vi "Process_calibration_test.vi"() -> ()   [LabVIEW 2015]
uses:
  <vilib>/Analysis/5stat.llb/RMS (DBL).vi
  <vilib>/measure/madcrms.llb/Basic Averaged DC-RMS for 1 Chan.vi
  <vilib>/measure/maspectr.llb/FFT Spectrum (Mag-Phase) for 1 Chan.vi
  <vilib>/measure/NI_MAPro.lvlib
  <vilib>/Analysis/NI_AALPro.lvlib
  <vilib>/Analysis/NI_AALBase.lvlib
  <vilib>/Analysis/3filter.llb/Butterworth Filter (DBL).vi
  <vilib>/Analysis/3filter.llb/Filter Passband Type.ctl
panel:
  out "Waveform Graph 4":waveform(dbl)[](graph)
  out "Calibration\nparameter":dbl
  out "Sensivity\ncalibrated\nmV/g":dbl
  in  "Pattern\namplitude":dbl=1.02
  out "Array 8":bool[](array[boolean])
  out "Mean\nfrequency":dbl format="%0.2f"
  out "Main\nFrequency":dbl[](array[numeric])
  out "Valid\nmeasur\nfrequency":bool[](array[boolean])
  out "max value 3":dbl
  out "max value 2":dbl
  out "x/y 2":dbl
  out "x/y":dbl
  out "max value":dbl
  out "max index(es)":i32
  out "df":dbl
  out "magnitude":dbl[](array[numeric])
  out "Waveform Graph 3":T1(graph)
  out "Array 7":dbl[](array[numeric])
  out "Array 6":bool[][](array[boolean])
  out "mV":dbl[][](array[numeric])
  out "Valid \nmeasurements":sgl[][](array[numeric])
  out "Valid index":dbl format="%0.2f"
  out "Array 5":bool[](array[boolean])
  out "x > y?":bool
  out "concatenated string":string
  out "Index\ninvalid":i32[](array[numeric])
  out "Valid\nindex 2":i32[](array[numeric])
  out "Nº meas.":i32
  out "Valid\nindex":i32[](array[numeric])
  out "Array 4":bool[](array[boolean])
  out "Array 2":i32[][](array[numeric])
  out "Array 3":i32[](array[numeric])
  out "All Files in Dir":path[](array[path])
  out "Array":bool[][](array[boolean])
  in  "Frecuencia\nmuestreo":dbl=25600.0
  in  "Pattern frequency (Hz)":dbl=159.2
  in  "Nº canales":i32=10
  out "Waveform Graph":waveform(dbl)[](graph)
  in  "Folder Path":path
  out "error out":errorcluster
  # "Min"
  # "Median"
  # "Mean"
  # "Variance"
  # "Max"
  # "G:\\Mi unidad\\WRD\\SERVICIOS_Disco_duro\\Euskotren\\Lugaritz\\2016-05\\Calibracion\\4D\\verde"
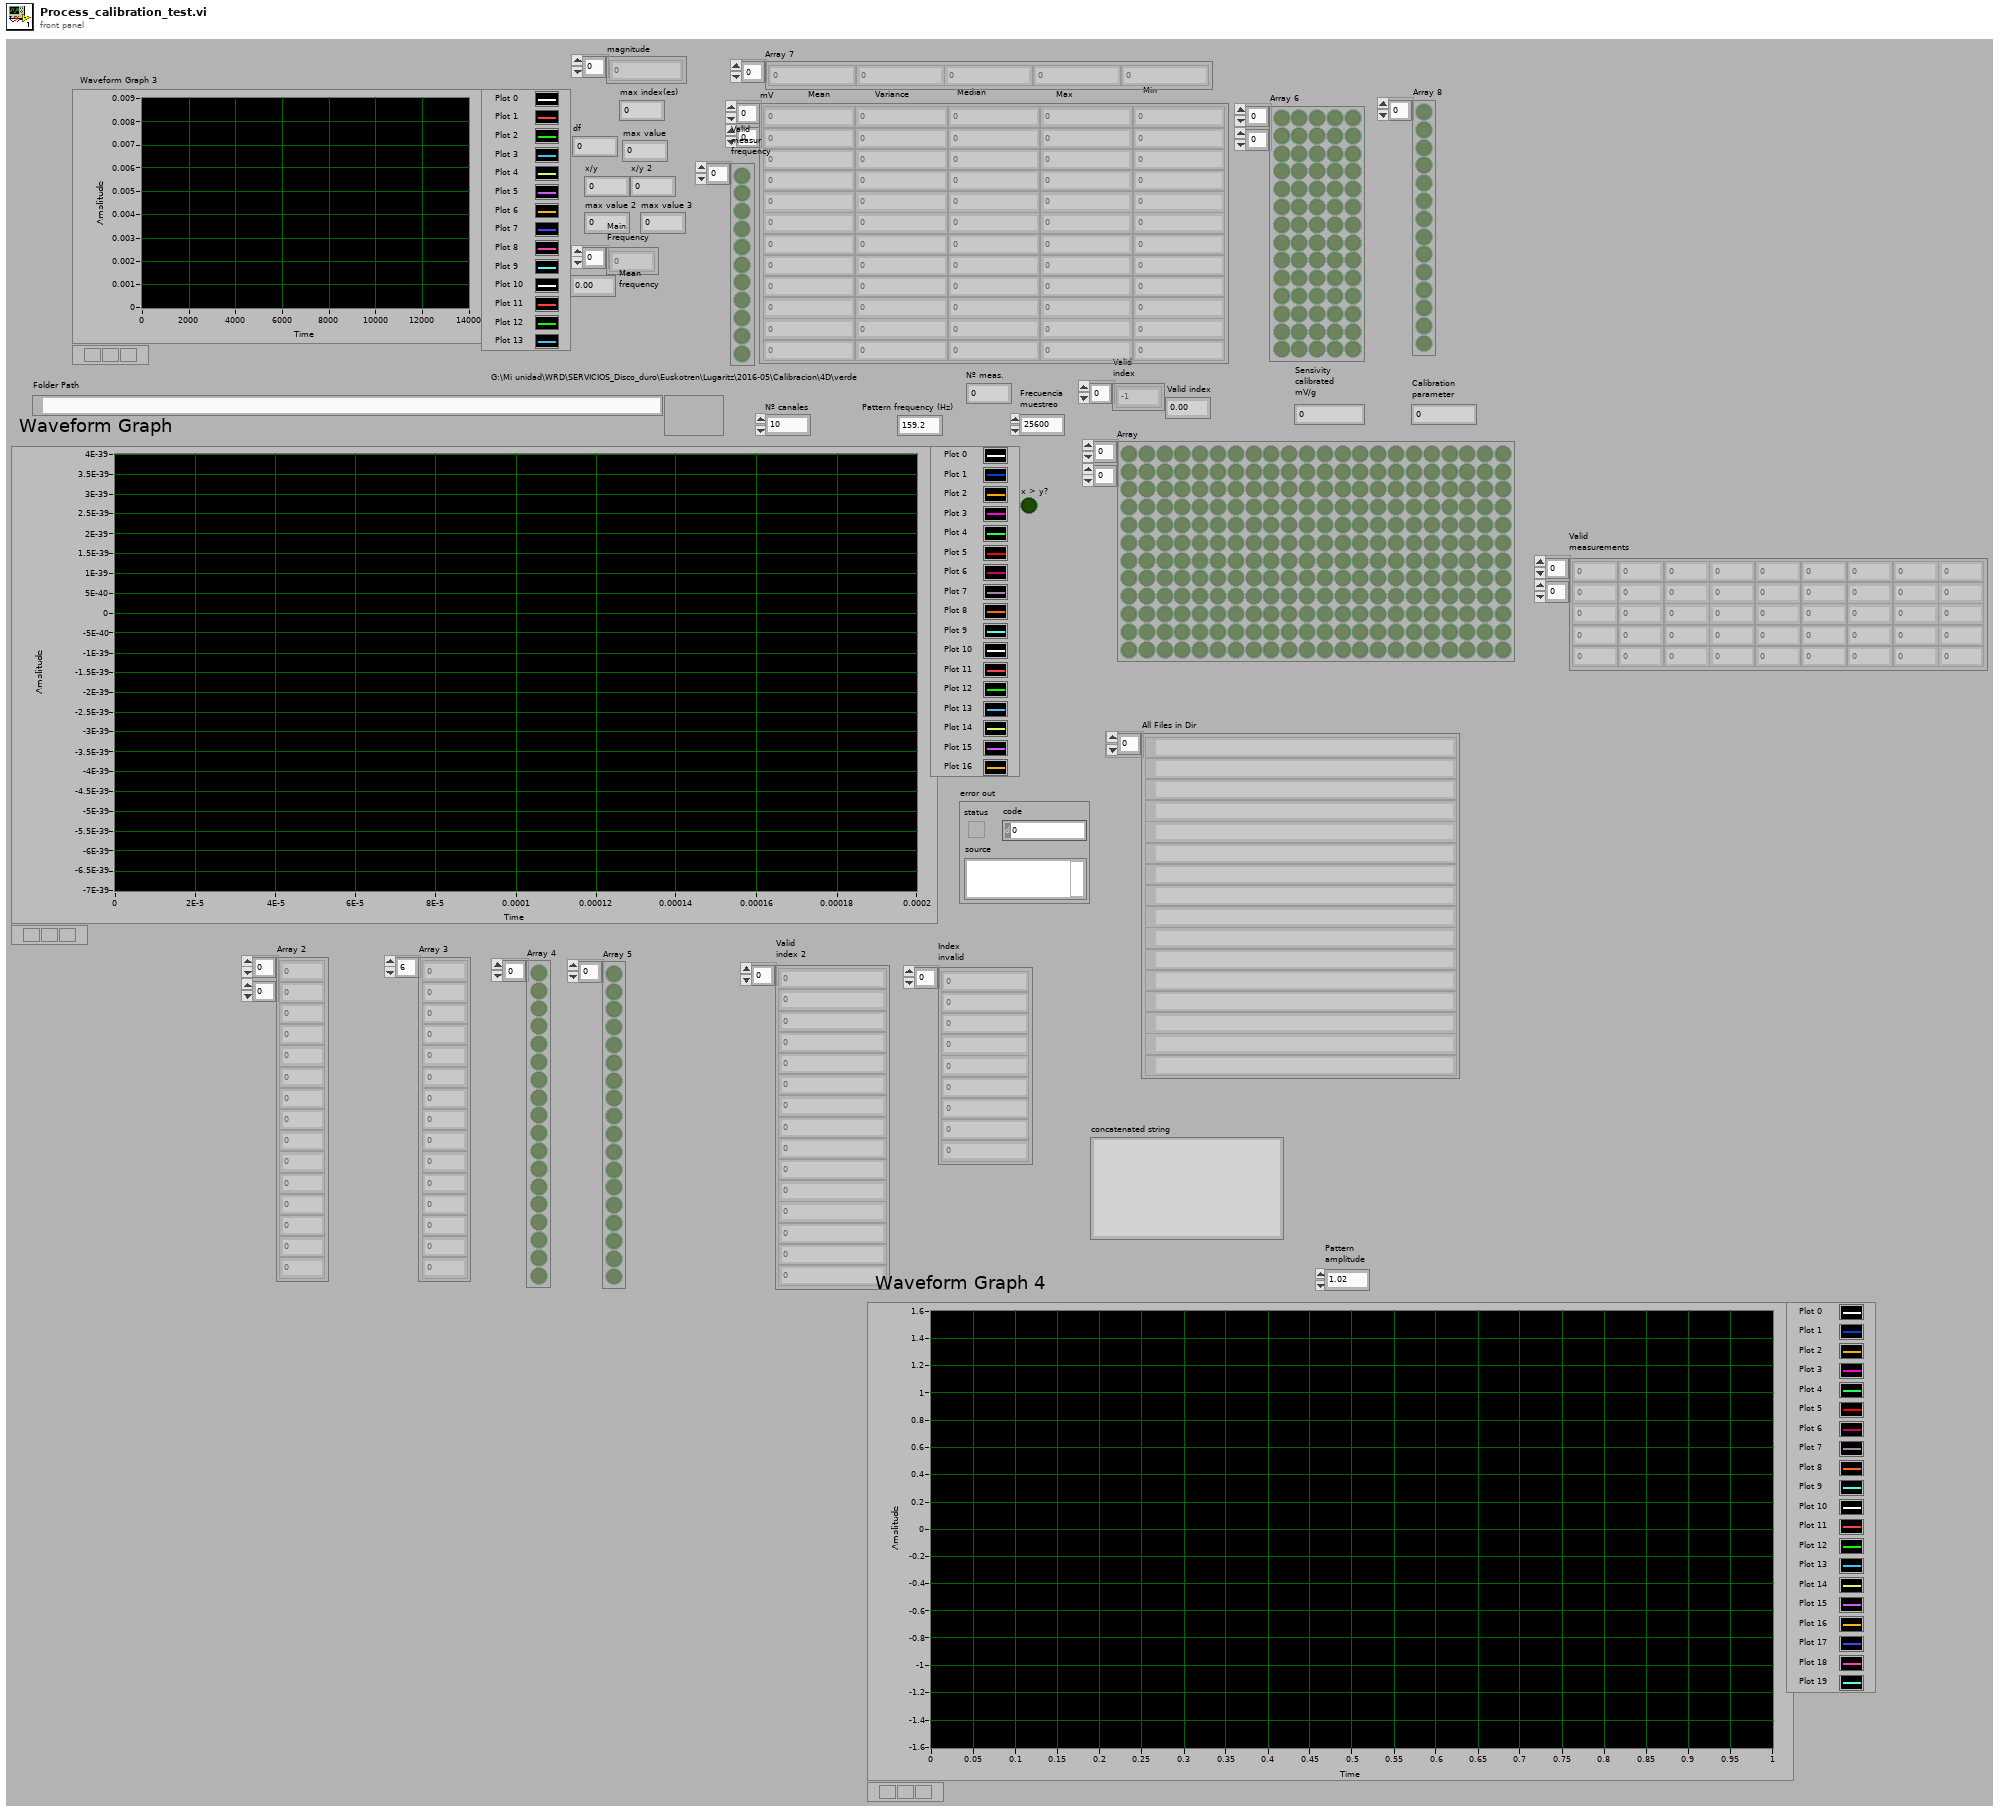
[diagram p1: front panel]
types:
  T1 = cluster{"f0":dbl, "df":dbl, "imaginary part":dbl[]}[]
  T2 = enum16{"big-endian, network order", "native, host order", "little-endian"}
  T3 = typedef "NI_AALBase.lvlib/Filter Passband Type.ctl" = enum32{"Lowpass", "Highpass", "Bandpass", "Bandstop"}
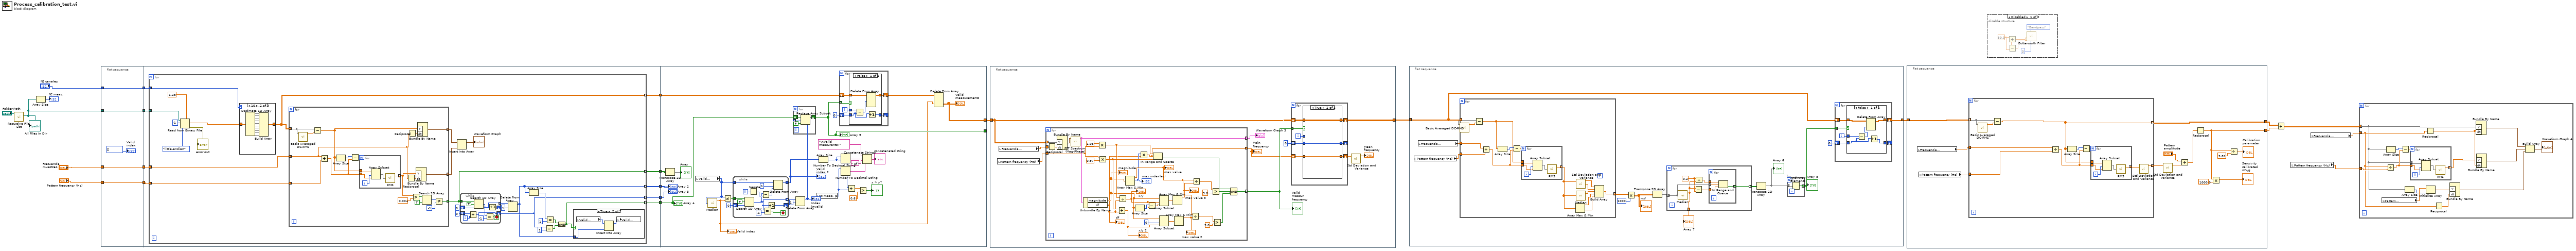
[diagram p0: block diagram]
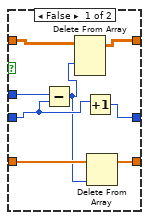
[diagram p3: hidden frame]
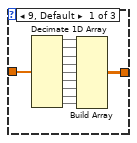
[diagram p6: hidden frame]
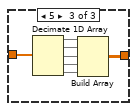
[diagram p7: hidden frame]
diagram:
  n1 = call <vilib>:"Recursive File List.vi"("Folder Path"="Folder Path") -> ("All Files in Dir"=w8:path[])  [unwired: 6 in, 4 out]
  "All Files in Dir" <- w8
  n2 = Array Size(array=w8) -> (size(s)=→"Nº meas.":i32)
  n3 = flat-sequence {
    tunnel: w8 -> [w27]
    tunnel: [w27] -> w7
    tunnel: [w26] -> w6
    tunnel: "Nº canales" -> [w26]
    tunnel: [w25] -> w4
    tunnel: "Frecuencia\nmuestreo" -> [w25]
    tunnel: [w24] -> w2
    tunnel: "Pattern frequency (Hz)" -> [w24]
    tunnel: [w36] -> w23
    tunnel: [w35] -> w22
    tunnel: [w34] -> w21
    tunnel: [w33] -> w20
    tunnel: [w32] -> w19
    tunnel: w7 -> [w37]
    tunnel: w6 -> [w31]
    tunnel: w4 -> [w30]
    tunnel: w2 -> [w29]
    tunnel: w23 -> [w158]
    tunnel: w22 -> [w155]
    tunnel: w21 -> [w156]
    tunnel: w20 -> [w137]
    tunnel: w19 -> [w136]
    tunnel: [w135] -> _
    tunnel: [w134] -> w18
    frame #0 {
      "Valid\nindex" <- i32[] []
    }
    frame #1 {
      n4 = for {
        tunnel: w37 -> [w55] mode=indexing
        tunnel: [w52] -> w36 mode=indexing
        tunnel: [w43] -> w35 mode=indexing
        tunnel: [w42] -> w34 mode=indexing
        tunnel: [w44] -> w33 mode=indexing
        tunnel: [w41] -> w32 mode=indexing
        tunnel: w31 -> [w40]
        tunnel: w30 -> [w39]
        tunnel: w29 -> [w38]
        n5 = Read from Binary File(5:sgl 1.25, 9:T2."little-endian" ("byte order (0:big-endian, network order)"), 10:-1 ("count (1)"), 11:w55) -> (0:→"error out":errorcluster, 2:w59:sgl[])  [unwired: 1 in, 3 out]
        n6 = case shown="10" w40 {
          tunnel: [w77 w90 w100] -> w41
          tunnel: w59 -> [w78 w88 w101]
          frame 9, Default {
            n7 = Decimate 1D Array(w78) -> (w79:sgl[], w87:sgl[], w86:sgl[], w82:sgl[], w81:sgl[], w83:sgl[], w84:sgl[], w85:sgl[], w80:sgl[])
            n8 = Build Array(w79, w87, w86, w82, w81, w83, w84, w85, w80) -> (w77:sgl[][])
          }
          frame 10 {
            n9 = Decimate 1D Array(w88) -> (w89:sgl[], w99:sgl[], w98:sgl[], w94:sgl[], w93:sgl[], w95:sgl[], w96:sgl[], w97:sgl[], w92:sgl[], w91:sgl[])
            n10 = Build Array(w89, w99, w98, w94, w93, w95, w96, w97, w92, w91) -> (w90:sgl[][])
          }
          frame 5 {
            n11 = Decimate 1D Array(w101) -> (w102:sgl[], w106:sgl[], w105:sgl[], w104:sgl[], w103:sgl[])
            n12 = Build Array(w102, w106, w105, w104, w103) -> (w100:sgl[][])
          }
        }
        n13 = for {
          tunnel: w41 -> [w123] mode=indexing
          tunnel: [w117] -> w58 mode=indexing
          tunnel: [w116] -> w57 mode=indexing
          tunnel: [w109] -> w52 mode=indexing
          tunnel: w39 -> [w108]
          tunnel: w38 -> [w107]
          n14 = call-poly <vilib>:"Basic Averaged DC-RMS.vi"("signal in"=w123) -> ("DC value"=w124:dbl)  [unwired: 7 in, 3 out]
          n15 = Subtract(x=w123, y=w124) -> (x-y=w118:dbl[])
          n16 = Divide(x=w108, y=w107) -> (x/y=w120:dbl)
          n17 = Array Size(array=w118) -> (size(s)=w121:i32)
          n18 = Subtract(x=w121, y=w120) -> (x-y=w122:dbl)
          n19 = for {
            N: w122 -> [_]
            tunnel: w120 -> [w127]
            tunnel: [w130] -> w115 mode=indexing
            tunnel: w118 -> [w129]
            i -> [w128]
            n20 = Array Subset(array=w129, index=w128, length=w127) -> (w126:dbl[])
            n21 = call-poly <vilib>:"RMS.vi"("X"=w126) -> ("rms value"=w130:dbl)  [unwired: 1 out]
          }
          n22 = Reciprocal(x=w108) -> (1/x=w119:dbl)
          n23 = Reciprocal(x=w108) -> (1/x=w125:dbl)
          n24 = Greater?(x=w115, y=0.004 ("threshold y")) -> (0:w113:bool[])
          n25 = Bundle By Name("Y"=w115, "dt"=w119) -> (w116:waveform(dbl))  [unwired: 1 in]
          n26 = Bundle By Name("Y"=w118, "dt"=w125) -> (w117:waveform(dbl))  [unwired: 1 in]
          n27 = Search 1D Array(1D array=w113, element=TRUE) -> (index of element=w111:i32)  [unwired: 1 in]
          n28 = Not Equal?(x=w111, y=-1) -> (x != y?=w109:bool)
        }
        n29 = Insert Into Array(array=w58, new element=w57) -> (→"Waveform Graph":waveform(dbl)[])  [unwired: 1 in]
        n30 = while {
          tunnel: w52 -> [w76]
          shift-right: [w68] -> _
          shift-left: 0 ("index of element") -> [w73]
          shift-right: [w69] -> w43
          shift-left: 0 ("index of element") -> [w70]
          tunnel: [w67] -> w50 mode=indexing
          i -> [w71]
          stop <- w74 stop-if-true
          n31 = Add(x=w70, y=w71) -> (x+y=w69:i32)
          n32 = Search 1D Array(1D array=w76, element=TRUE, start index (0)=w73) -> (index of element=w67:i32)
          n33 = Equal?(x=w67, y=-1) -> (x = y?=w74:bool)
          n34 = Increment(x=w67) -> (x+1=w68:i32)
        }
        n35 = Delete From Array(array=w50, length=1) -> (array with subset deleted=w42:i32[])  [unwired: 1 in, 1 out]
        n36 = Array Size(array=w42) -> (size(s)=w47:i32)
        n37 = Equal?(x=w43, y=1) -> (x = y?=w46:bool)
        n38 = Equal?(x=w47, y=1) -> (x = y?=w45:bool)
        n39 = And(x=w45, y=w46) -> (x .and. y?=w44:bool)
        n40 = case shown="True" w44 {
          tunnel: w42 -> [_ w64]
          frame False {
          }
          frame True {
            n41 = local read "Valid\nindex"() -> (w66:i32[])
            n42 = Insert Into Array(array=w66, new element=w64) -> (w65:i32[])  [unwired: 1 in]
            n43 = local write "Valid\nindex"(w65) -> ()
          }
        }
      }
    }
    frame #2 {
      n44 = Transpose 2D Array(2D array=w158) -> (transposed array=→"Array":bool[][])
      n45 = local read "Valid\nindex"() -> (w153:i32[])
      n46 = call <vilib>:"Median.vi"("X"=w153) -> ("median"=w131:dbl)  [unwired: 1 out]
      "Valid index" <- w131
      n47 = Not Equal?(x=w153, y=w131) -> (x != y?=w154:bool[])
      n48 = while {
        tunnel: w154 -> [w189]
        tunnel: w153 -> [w183]
        shift-right: [w185] -> _
        shift-left: 0 ("index of element") -> [w184]
        tunnel: [w178] -> w149
        tunnel: [w177] -> w151 mode=indexing
        i -> [w181]
        stop <- w186 stop-if-true
        n49 = Search 1D Array(1D array=w189, element=TRUE, start index (0)=w184) -> (index of element=w177:i32)
        n50 = Negate(x=w181) -> (-x=w180:i32)
        n51 = Subtract(x=w177, y=w180) -> (x-y=w179:i32)
        n52 = Equal?(x=w177, y=-1) -> (x = y?=w186:bool)
        n53 = Increment(x=w177) -> (x+1=w185:i32)
        n54 = Delete From Array(array=w183, length=1, index=w179) -> (array with subset deleted=w178:i32[])  [unwired: 1 out]
      }
      "Valid\nindex 2" <- w149
      n55 = Delete From Array(array=w151, length=1) -> (array with subset deleted=w138:i32[])  [unwired: 1 in, 1 out]
      "Index\ninvalid" <- w138
      n56 = for {
        tunnel: w138 -> [w176] mode=indexing
        shift-right: [w174] -> w135
        shift-left: w137 -> [w173]
        n57 = Replace Array Subset(array=w173, new element=FALSE ("new element/subarray"), index=w176) -> (w174:bool[])
      }
      "Array 5" <- w135
      n58 = local read "Nº meas."() -> (w142:i32)
      n59 = Array Size(array=w149) -> (size(s)=w143:i32)
      n60 = for {
        tunnel: w135 -> [w163] mode=indexing
        shift-right: [w162] -> w133
        shift-left: w136 -> [w164]
        shift-right: [w159] -> _
        shift-left: 0 ("index of element") -> [w160]
        i -> [w161]
        n61 = case shown="False" w163 {
          tunnel: w164 -> [w170 w172]
          tunnel: [w169 w172] -> w162
          tunnel: w161 -> [w168 _]
          tunnel: w160 -> [w165 w171]
          tunnel: [w166 w171] -> w159
          frame False {
            n62 = Subtract(x=w168, y=w165) -> (x-y=w167:i32)
            n63 = Delete From Array(array=w170, index (dim 0)=w167) -> (array with subset deleted=w169:sgl[][][])  [unwired: 3 in, 1 out]
            n64 = Increment(x=w165) -> (x+1=w166:i32)
          }
          frame True {
          }
        }
      }
      n65 = Number To Decimal String(number=w143) -> (decimal integer string=w147:string)  [unwired: 1 in]
      n66 = Number To Decimal String(number=w142) -> (decimal integer string=w145:string)  [unwired: 1 in]
      n67 = Divide(x=w143, y=w142) -> (x/y=w141:dbl)
      n68 = Greater?(x=w141, y=0.6) -> (0:→"x > y?":bool)
      n69 = Concatenate Strings("\nValid measurents: ", w147, " of ", w145) -> (→"concatenated string":string)
      n70 = Delete From Array(array=w133, index (dim 1)=w131) -> (deleted portion=w134:sgl[][])  [unwired: 3 in, 1 out]
      "Valid \nmeasurements" <- w134
      "Array 3" <- w155
      "Array 2" <- w156
      "Array 4" <- w137
    }
  }
  n71 = flat-sequence {
    tunnel: w18 -> [w194]
    tunnel: [w196] -> w17
    frame #0 {
      n72 = local read "Pattern frequency (Hz)"() -> (w197:dbl)
      n73 = local read "Frecuencia\nmuestreo"() -> (w199:dbl)
      n74 = for {
        tunnel: w194 -> [w249] mode=indexing
        tunnel: w199 -> [w248]
        tunnel: [w246] -> w198 mode=indexing
        tunnel: w197 -> [w244]
        tunnel: [w225] -> w193 mode=indexing
        tunnel: [w219] -> w192 mode=indexing
        n75 = Reciprocal(x=w248) -> (1/x=w250:dbl)
        n76 = Bundle By Name("Y"=w249, "dt"=w250) -> (w247:waveform(sgl))  [unwired: 1 in]
        n77 = call-poly <vilib>:"FFT Spectrum (Mag-Phase).vi"("time signal"=w247) -> ("magnitude"=w246:cluster{"f0":dbl, "df":dbl, "magnitude":dbl[]})  [unwired: 6 in, 4 out]
        n78 = Unbundle By Name(w246) -> ("magnitude"=w238:dbl[], "df"=w220:dbl)
        "magnitude" <- w238
        "df" <- w220
        n79 = Multiply(x=1.03, y=w244) -> (x*y=w241:dbl)
        n80 = Multiply(x=w244, y=0.97 ("x")) -> (x*y=w242:dbl)
        n81 = Divide(x=w242, y=w220) -> (x/y=w239:dbl)
        "x/y 2" <- w239
        n82 = Divide(x=w241, y=w220) -> (x/y=w236:dbl)
        "x/y" <- w236
        n83 = Array Max & Min(array=w238) -> (max value=w231:dbl, max index (indices)=w221:i32)  [unwired: 2 out]
        "max index(es)" <- w221
        "max value" <- w231
        n84 = Array Size(array=w238) -> (size(s)=w237:i32)
        n85 = Multiply(x=w221, y=w220) -> (x*y=w219:dbl)
        n86 = Subtract(x=w237, y=w236) -> (x-y=w235:dbl)
        n87 = In Range and Coerce(upper limit=w241, x=w219, lower limit=w242) -> (In Range?=w224:bool)  [unwired: 1 out]
        n88 = Array Subset(array=w238, index=w236, length=w235) -> (w234:dbl[])
        n89 = Array Subset(array=w238, index=0, length=w239) -> (w233:dbl[])
        n90 = Array Max & Min(array=w234) -> (max value=w232:dbl)  [unwired: 3 out]
        "max value 3" <- w232
        n91 = Array Max & Min(array=w233) -> (max value=w230:dbl)  [unwired: 3 out]
        "max value 2" <- w230
        n92 = Divide(x=w231, y=w230) -> (x/y=w228:dbl)
        n93 = Divide(x=w231, y=w232) -> (x/y=w229:dbl)
        n94 = Greater?(x=w229, y=3.0) -> (0:w223:bool)
        n95 = Greater?(x=w228, y=3.0) -> (0:w222:bool)
        n96 = Compound Arithmetic op=AND(w224, w223, w222) -> (w225:bool)
      }
      "Waveform Graph 3" <- w198
      "Valid\nmeasur\nfrequency" <- w193
      "Main\nFrequency" <- w192
      n97 = for {
        shift-right: [w206] -> w196
        shift-left: w194 -> [w207]
        tunnel: w193 -> [w205] mode=indexing
        shift-right: [w202] -> _
        shift-left: 0 ("index of element") -> [w203]
        shift-right: [w200] -> w191
        shift-left: w192 -> [w201]
        i -> [w204]
        n98 = case shown="True" w205 {
          tunnel: w207 -> [w215 w218]
          tunnel: [w214 w218] -> w206
          tunnel: w204 -> [w213 _]
          tunnel: w203 -> [w212 w217]
          tunnel: [w211 w217] -> w202
          tunnel: w201 -> [w210 w216]
          tunnel: [w208 w216] -> w200
          frame False {
            n99 = Subtract(x=w213, y=w212) -> (x-y=w209:i32)
            n100 = Delete From Array(array=w215, index (row)=w209) -> (array with subset deleted=w214:sgl[][])  [unwired: 2 in, 1 out]
            n101 = Increment(x=w212) -> (x+1=w211:i32)
            n102 = Delete From Array(array=w210, index=w209) -> (array with subset deleted=w208:dbl[])  [unwired: 1 in, 1 out]
          }
          frame True {
          }
        }
      }
      n103 = call <vilib>:"Std Deviation and Variance.vi"("X"=w191) -> ("mean"=→"Mean\nfrequency":dbl)  [unwired: 1 in, 2 out]
    }
  }
  n104 = flat-sequence {
    tunnel: w17 -> [w252]
    tunnel: [w251] -> w16
    frame #0 {
      n105 = local read "Pattern frequency (Hz)"() -> (w256:dbl)
      n106 = local read "Frecuencia\nmuestreo"() -> (w257:dbl)
      n107 = for {
        tunnel: w252 -> [w303] mode=indexing
        tunnel: [w296] -> w263 mode=indexing
        tunnel: w257 -> [w290]
        tunnel: w256 -> [w291]
        n108 = call-poly <vilib>:"Basic Averaged DC-RMS.vi"("signal in"=w303) -> ("DC value"=w304:dbl)  [unwired: 7 in, 3 out]
        n109 = Subtract(x=w303, y=w304) -> (x-y=w292:dbl[])
        n110 = Divide(x=w290, y=w291) -> (x/y=w300:dbl)
        n111 = Array Size(array=w292) -> (size(s)=w301:i32)
        n112 = Subtract(x=w301, y=w300) -> (x-y=w302:dbl)
        n113 = for {
          N: w302 -> [_]
          tunnel: w300 -> [w306]
          tunnel: [w309] -> w293 mode=indexing
          tunnel: w292 -> [w308]
          i -> [w307]
          n114 = Array Subset(array=w308, index=w307, length=w306) -> (w305:dbl[])
          n115 = call-poly <vilib>:"RMS.vi"("X"=w305) -> ("rms value"=w309:dbl)  [unwired: 1 out]
        }
        n116 = Array Max & Min(array=w293) -> (max value=w298:dbl, min value=w297:dbl)  [unwired: 2 out]
        n117 = call <vilib>:"Std Deviation and Variance.vi"("X"=w293) -> ("mean"=w294:dbl, "standard deviation"=w295:dbl)  [unwired: 1 in, 1 out]
        n118 = call <vilib>:"Median.vi"("X"=w293) -> ("median"=w299:dbl)  [unwired: 1 out]
        n119 = Build Array(w294, w295, w299, w298, w297) -> (w296:dbl[])
      }
      n120 = Multiply(x=w263, y=1000 ("median")) -> (x*y=w259:dbl[][])
      "mV" <- w259
      n121 = Transpose 2D Array(2D array=w259) -> (transposed array=w260:dbl[][])
      n122 = for {
        tunnel: w260 -> [w285] mode=indexing
        tunnel: [w280] -> w258 mode=indexing
        tunnel: [w281] -> w261 mode=indexing
        w283 = 0.2 ("x")
        n123 = call <vilib>:"Median.vi"("X"=w285) -> ("median"=w281:dbl)  [unwired: 1 out]
        n124 = Subtract(x=w281, y=w283) -> (x-y=w282:dbl)
        n125 = Add(x=w283, y=w281) -> (x+y=w284:dbl)
        n126 = for {
          tunnel: w285 -> [w289] mode=indexing
          tunnel: w284 -> [w288]
          tunnel: w282 -> [w287]
          tunnel: [w286] -> w280 mode=indexing
          n127 = In Range and Coerce(upper limit=w288, x=w289, lower limit=w287) -> (In Range?=w286:bool)  [unwired: 1 out]
        }
      }
      "Array 7" <- w261
      n128 = Transpose 2D Array(2D array=w258) -> (transposed array=w255:bool[][])
      "Array 6" <- w255
      n129 = for {
        tunnel: w255 -> [w279] mode=indexing
        tunnel: [w278] -> w253 mode=indexing
        n130 = And Array Elements(Boolean array=w279) -> (logical AND=w278:bool)
      }
      "Array 8" <- w253
      n131 = for {
        shift-right: [w268] -> w251
        shift-left: w252 -> [w269]
        tunnel: w253 -> [w267] mode=indexing
        shift-right: [w264] -> _
        shift-left: 0 ("index of element") -> [w265]
        i -> [w266]
        n132 = case shown="False" w267 {
          tunnel: w269 -> [w275 w277]
          tunnel: [w274 w277] -> w268
          tunnel: w266 -> [w273 _]
          tunnel: w265 -> [w272 w276]
          tunnel: [w271 w276] -> w264
          frame False {
            n133 = Subtract(x=w273, y=w272) -> (x-y=w270:i32)
            n134 = Delete From Array(array=w275, index (row)=w270) -> (array with subset deleted=w274:sgl[][])  [unwired: 2 in, 1 out]
            n135 = Increment(x=w272) -> (x+1=w271:i32)
          }
          frame True {
          }
        }
      }
    }
  }
  n136 = flat-sequence {
    tunnel: w16 -> [w314]
    tunnel: [w313] -> w15
    tunnel: [w310] -> w14
    frame #0 {
      n137 = local read "Frecuencia\nmuestreo"() -> (w322:dbl)
      n138 = local read "Pattern frequency (Hz)"() -> (w321:dbl)
      n139 = for {
        tunnel: w314 -> [w331] mode=indexing
        tunnel: w322 -> [w327]
        tunnel: w321 -> [w324]
        tunnel: [w325] -> w320 mode=indexing
        tunnel: [w323] -> w313 mode=indexing
        n140 = call-poly <vilib>:"Basic Averaged DC-RMS.vi"("signal in"=w331) -> ("DC value"=w332:dbl)  [unwired: 7 in, 3 out]
        n141 = Subtract(x=w331, y=w332) -> (x-y=w323:dbl[])
        n142 = Divide(x=w327, y=w324) -> (x/y=w328:dbl)
        n143 = Array Size(array=w323) -> (size(s)=w329:i32)
        n144 = Subtract(x=w329, y=w328) -> (x-y=w330:dbl)
        n145 = for {
          N: w330 -> [_]
          tunnel: w328 -> [w334]
          tunnel: [w337] -> w326 mode=indexing
          tunnel: w323 -> [w336]
          i -> [w335]
          n146 = Array Subset(array=w336, index=w335, length=w334) -> (w333:dbl[])
          n147 = call-poly <vilib>:"RMS.vi"("X"=w333) -> ("rms value"=w337:dbl)  [unwired: 1 out]
        }
        n148 = call <vilib>:"Std Deviation and Variance.vi"("X"=w326) -> ("mean"=w325:dbl)  [unwired: 1 in, 2 out]
      }
      n149 = call <vilib>:"Std Deviation and Variance.vi"("X"=w320) -> ("mean"=w319:dbl)  [unwired: 1 in, 2 out]
      n150 = Divide(x="Pattern\namplitude", y=w319) -> (x/y=w316:dbl)
      n151 = Reciprocal(x=w316) -> (1/x=w310:dbl)
      n152 = Multiply(x=w310, y=1000.0) -> (x*y=→"Sensivity\ncalibrated\nmV/g":dbl)
      n153 = Divide(x=w310, y=9.81) -> (x/y=→"Calibration\nparameter":dbl)
    }
  }
  n154 = disable-structure shown="Disabled" {
    frame Disabled {
      w343 = 50.0 ("y")
      n155 = Add(x=w343) -> (y=w338:dbl, x+y=w344:dbl)
      n156 = Subtract(x=w338, y=w343) -> (x-y=w345:dbl)
      n157 = call-poly <vilib>:"Butterworth Filter.vi"("order"=3, "filter type"=Filter_Passband_Type."Bandpass", "low cutoff freq: fl"=w345, "high cutoff freq: fh"=w344) -> ("sampling freq: fs"=w339:dbl, "X"=w340:dbl[])  [unwired: 2 in, 2 out]
    }
    frame Enabled {
    }
  }
  n158 = Divide(x=w15, y=w14) -> (x/y=w13:dbl[][])
  n159 = local read "Pattern frequency (Hz)"() -> (w12:dbl)
  n160 = local read "Frecuencia\nmuestreo"() -> (w11:dbl)
  n161 = for {
    tunnel: w13 -> [w347] mode=indexing
    tunnel: w12 -> [w359]
    tunnel: w11 -> [w349]
    n162 = local read "Pattern\namplitude"() -> (w352:dbl)
    n163 = Divide(x=w349, y=w359) -> (x/y=w358:dbl)
    n164 = Array Size(array=w347) -> (size(s)=w360:i32)
    n165 = Subtract(x=w360, y=w358) -> (x-y=w361:dbl)
    n166 = Array Size(array=w347) -> (size(s)=w351:i32)
    n167 = for {
      N: w361 -> [_]
      tunnel: w358 -> [w363]
      tunnel: [w366] -> w346 mode=indexing
      tunnel: w347 -> [w365]
      i -> [w364]
      n168 = Array Subset(array=w365, index=w364, length=w363) -> (w362:dbl[])
      n169 = call-poly <vilib>:"RMS.vi"("X"=w362) -> ("rms value"=w366:dbl)  [unwired: 1 out]
    }
    n170 = Reciprocal(x=w349) -> (1/x=w357:dbl)
    n171 = Initialize Array(w352, w351) -> (w350:dbl[])
    n172 = Reciprocal(x=w349) -> (1/x=w353:dbl)
    n173 = Bundle By Name("Y"=w350, "dt"=w353) -> (w348:waveform(dbl))  [unwired: 1 in]
    n174 = Bundle By Name("Y"=w347, "dt"=w357) -> (w355:waveform(dbl))  [unwired: 1 in]
    n175 = Bundle By Name("Y"=w346, "dt"=w357) -> (w354:waveform(dbl))  [unwired: 1 in]
    n176 = Build Array(w355, w354, w348) -> (→"Waveform Graph 4":waveform(dbl)[])
  }
